vi "Read FPGA.vi"(8 "error in (no error)":errorcluster, 11 "Run Instance in":refnum<class "Run Instance.lvclass">) -> (0 "error out":errorcluster, 2 "FPGA Name":string, 3 "Run Instance out":refnum<class "Run Instance.lvclass">)   [LabVIEW 2020, in "CIRCUS_uServices.lvlib" / "Run Utilities.lvlib" / "Run Instance.lvclass"]
uses:
  Run Instance.lvclass
  Run Instance.lvclass/Run Instance.ctl
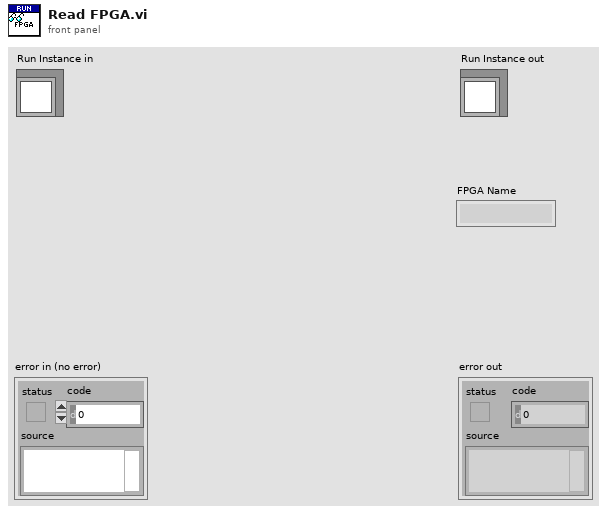
[diagram p1: front panel]
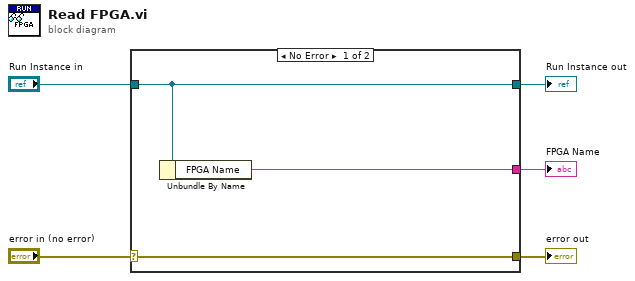
[diagram p0: block diagram]
diagram:
  n1 = case shown="No Error" "error in (no error)" {
    selector: "error in (no error)" -> [w8 w9]
    tunnel: [w8 w9] -> w4
    tunnel: [w7 w10] -> w2
    tunnel: "Run Instance in" -> [w7 w10]
    tunnel: [w6 _] -> w1
    frame No Error {
      n2 = Unbundle By Name(w7) -> ("FPGA Name"=w6:string)
    }
    frame Error {
    }
  }
  "error out" <- w4
  "Run Instance out" <- w2
  "FPGA Name" <- w1
